vi "Task Config.vi"(8 "error in (no error)":errorcluster, 11 "Module in":refnum<class "Module.lvclass">) -> (0 "error out":errorcluster, 2 "Task Config":refnum<class "Task.lvclass">, 3 "Module out":refnum<class "Module.lvclass">)   [LabVIEW 2020, in "Volatus.lvlib" / "Module.lvclass"]
uses:
  Module.lvclass
  Module.lvclass/Module.ctl
  VolatusConfig/Task/Task.lvclass
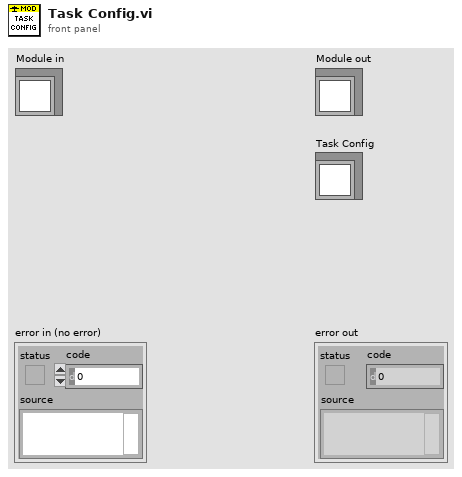
[diagram p1: front panel]
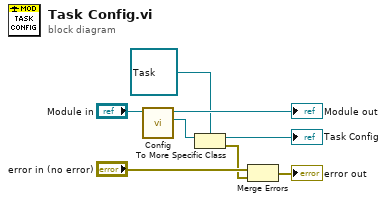
[diagram p0: block diagram]
diagram:
  n1 = call "Config.vi"("Module in"="Module in") -> ("Config"=w5:refnum<class "VolatusConfigElement.lvclass">, "Module out"=→"Module out":refnum<class "Module.lvclass">)  [unwired: 9 in]
  n2 = To More Specific Class(target class=refnum<class "Task.lvclass"> refnum ("VolatusConfig.lvlib:Task.lvclass"), reference=w5) -> (specific class reference=→"Task Config":refnum<class "Task.lvclass">, error out=w1:errorcluster)  [unwired: 1 in]
  n3 = Merge Errors("error in (no error)", w1) -> (→"error out":errorcluster)
